vi "sum_minus_block.vi"(2 "Control":T3, 3 "B":T4, 4 "A":T5) -> (0 "Flags":T1, 1 "Result":T2)   [LabVIEW 2013]
panel:
  # "R1"
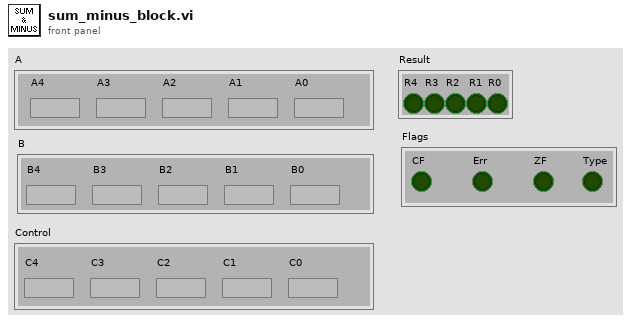
[diagram p1: front panel]
types:
  T1 = cluster{"CF":bool, "Err":bool, "ZF":bool, "Type":bool}
  T2 = cluster{"R4":bool, "R3":bool, "R2":bool, bool, "R0":bool}
  T3 = cluster{"C4":bool, "C3":bool, "C2":bool, "C1":bool, "C0":bool}
  T4 = cluster{"B4":bool, "B3":bool, "B2":bool, "B1":bool, "B0":bool}
  T5 = cluster{"A4":bool, "A3":bool, "A2":bool, "A1":bool, "A0":bool}
  T6 = cluster{"Y5":bool, "Y4":bool, "Y3":bool, "Y2":bool, "Y1":bool, "Y0":bool}
  T7 = cluster{"Y4":bool, "Y3":bool, "Y2":bool, "Y1":bool, "Y0":bool}
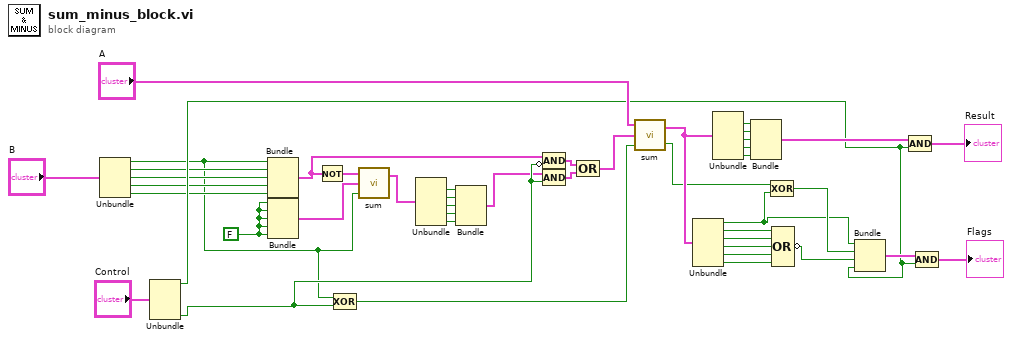
[diagram p0: block diagram]
diagram:
  w3 = FALSE
  n1 = Unbundle("B") -> ("B4"=w1:bool, "B3"=w22:bool, "B2"=w21:bool, "B1"=w20:bool, "B0"=w19:bool)
  n2 = Unbundle("Control") -> ("C4"=w25:bool, "C0"=w14:bool)  [unwired: 3 out]
  n3 = Bundle("B4"=w1, "B3"=w22, "B2"=w21, "B1"=w20, "B0"=w19) -> (w15:T4)  [unwired: 1 in]
  n4 = Bundle(w3, w3, w3, w3, w3) -> (w2:cluster{bool, bool, bool, bool, bool})  [unwired: 1 in]
  n5 = Not(x=w15) -> (.not. x?=w11:T4)
  n6 = Compound Arithmetic op=XOR(w1, w14) -> (w23:bool)
  n7 = call "sum.vi"("+1"=w1, "B"=w2, "A"=w11) -> ("Output"=w10:T6)  [unwired: 1 out]
  n8 = Unbundle(w10) -> ("Y4"=w9:bool, "Y3"=w8:bool, "Y2"=w7:bool, "Y1"=w6:bool, "Y0"=w5:bool)  [unwired: 1 out]
  n9 = Bundle("Y4"=w9, "Y3"=w8, "Y2"=w7, "Y1"=w6, "Y0"=w5) -> (w4:T7)  [unwired: 1 in]
  n10 = Compound Arithmetic op=AND(w15, invert w14) -> (w17:T4)
  n11 = Compound Arithmetic op=AND(w4, w14) -> (w16:T7)
  n12 = Compound Arithmetic op=OR(w17, w16) -> (w18:cluster{bool, bool, bool, bool, bool})
  n13 = call "sum.vi"("+1"=w23, "B"=w18, "A"="A") -> ("C"=w13:bool, "Output"=w35:T6)
  n14 = Unbundle(w35) -> ("Y5"=w12:bool, "Y4"=w37:bool, "Y3"=w41:bool, "Y2"=w40:bool, "Y1"=w39:bool, "Y0"=w38:bool)
  n15 = Unbundle(w35) -> ("Y4"=w34:bool, "Y3"=w33:bool, "Y2"=w32:bool, "Y1"=w31:bool, "Y0"=w30:bool)  [unwired: 1 out]
  n16 = Bundle("Y4"=w34, "Y3"=w33, "Y2"=w32, "Y1"=w31, "Y0"=w30) -> (w26:T7)  [unwired: 1 in]
  n17 = Compound Arithmetic op=XOR(w13, w12) -> (w36:bool)
  n18 = Compound Arithmetic op=OR(w37, w41, w40, w39, w38) -> (invert w42:bool)
  n19 = Bundle("Y5"=w12, w36, w42, "C4"=w25) -> (w29:cluster{"Y5":bool, bool, bool, "C4":bool})  [unwired: 1 in]
  n20 = Compound Arithmetic op=AND(w26, w25) -> (→"Result":T7)
  n21 = Compound Arithmetic op=AND(w29, w25) -> (→"Flags":cluster{"Y5":bool, bool, bool, "C4":bool})
